vi "Cernox Temp.vi"() -> (2 "Initial Base Temperature":dbl format="%.2f")   [LabVIEW 2010]
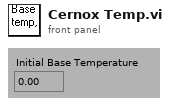
[diagram p1: front panel]
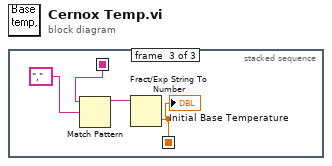
[diagram p0: block diagram]
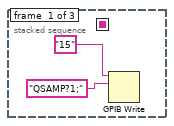
[diagram p2: hidden frame]
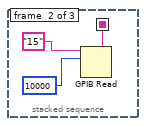
[diagram p3: hidden frame]
diagram:
  n1 = stacked-sequence {
    seq-local: [_ w3 _] -> [_ _ w9]
    seq-local: [_ _ w6] -> [_ _ _]
    frame #0 {
      n2 = GPIB Write(0:"15" ("address string"), 1:"QSAMP?1;" ("data")) -> ()  [unwired: 1 in, 4 out]
    }
    frame #1 {
      n3 = GPIB Read(0:"15" ("address string"), 1:10000 ("byte count")) -> (5:w3:string)  [unwired: 1 in, 4 out]
    }
    frame #2 {
      n4 = Match Pattern(string=w9, regular expression=",") -> (before substring=w7:string)  [unwired: 4 out]
      n5 = Fract/Exp String To Number(string=w7) -> (number=w6:dbl)  [unwired: 4 out]
      "Initial Base Temperature" <- w6
    }
  }
